vi "Refresh Display.vi"(6 "WaveformTemplate":waveform(dbl), 8 "error in":errorcluster, 9 "Temperature":dbl[](array[numeric]), 10 "Resistance":dbl[](array[numeric]), 11 "PRM in":refnum<class "PRM.lvclass">) -> (0 "error out":errorcluster, 2 "Measured":waveform(dbl)[](array[waveform]), 3 "PRM out":refnum<class "PRM.lvclass">)   [LabVIEW 2019, in "PRM.lvlib" / "PRM.lvclass"]
uses:
  Library/PRM.lvclass
  Library/PRM.lvclass/PRM.ctl
  builds/Instruments/Instruments.lvlibp/Library/Instruments.lvclass
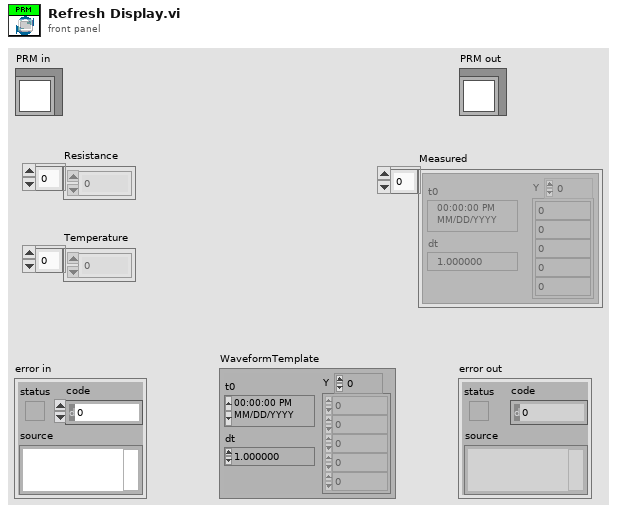
[diagram p1: front panel]
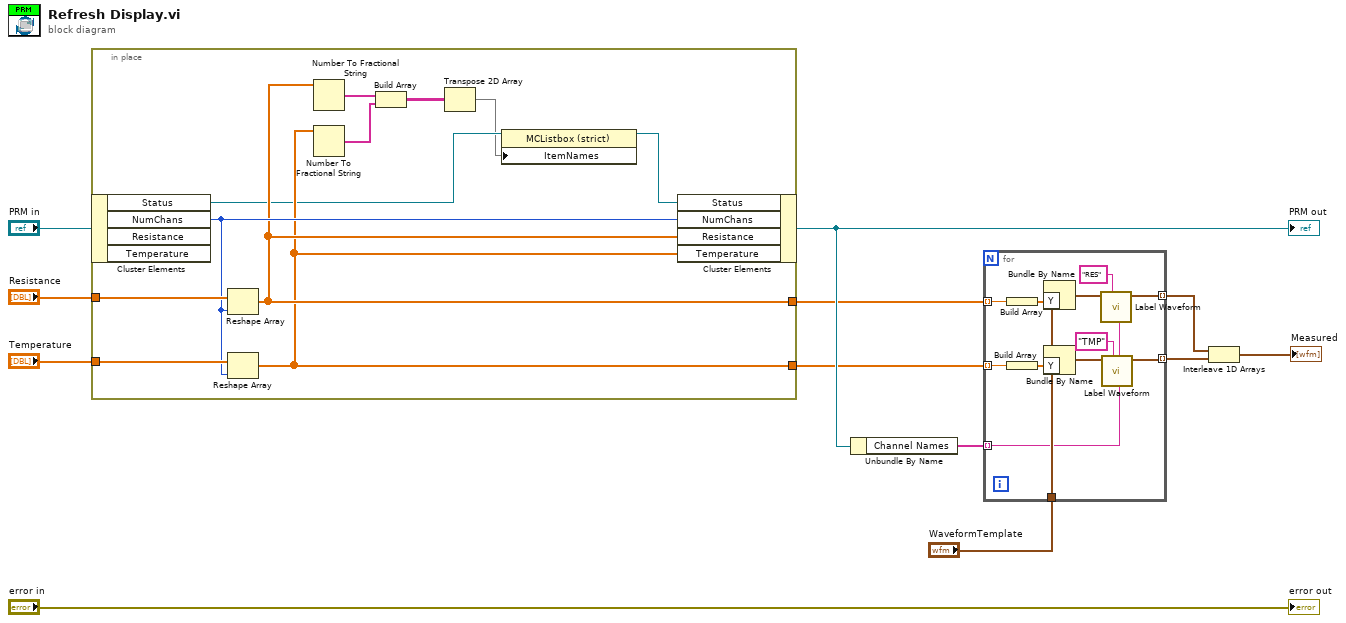
[diagram p0: block diagram]
diagram:
  n1 = in-place {
    in-place-border: "Resistance" -> [w23]
    in-place-border: "Temperature" -> [w22]
    in-place-border: [w20] -> w7
    in-place-border: [w19] -> w6
    n2 = in-place-cluster #1("PRM in") -> ("Status"=w16:refnum<vi>, "NumChans"=w21:i32)  [unwired: 2 out]
    n3 = Reshape Array(w23, w21) -> (w20:dbl[])
    n4 = Reshape Array(w22, w21) -> (w19:dbl[])
    n5 = Number To Fractional String(number=w20) -> (F-format string=w18:string[])  [unwired: 3 in]
    n6 = Number To Fractional String(number=w19) -> (F-format string=w17:string[])  [unwired: 3 in]
    n7 = Build Array(w18, w17) -> (w14:string[][])
    n8 = Transpose 2D Array(2D array=w14) -> (transposed array=w13:string[][])
    n9 = property class="MCListbox (strict)"(reference=w16, "ItemNames"=w13) -> (reference out=w15:refnum<vi>)  [unwired: 1 in, 1 out]
    n10 = in-place-cluster #1("Status"=w15, "NumChans"=w21, "Resistance"=w20, "Temperature"=w19) -> (w9:refnum<class "PRM.lvclass">)
  }
  "PRM out" <- w9
  n11 = Unbundle By Name(w9) -> ("Channel Names"=w8:string[])
  n12 = for {
    tunnel: w8 -> [w26] mode=indexing
    tunnel: w7 -> [w32] mode=indexing
    tunnel: w6 -> [w35] mode=indexing
    tunnel: "WaveformTemplate" -> [w31]
    tunnel: [w28] -> w3 mode=indexing
    tunnel: [w27] -> w2 mode=indexing
    n13 = Build Array(w32) -> (w33:dbl[])
    n14 = Build Array(w35) -> (w34:dbl[])
    n15 = Bundle By Name(cluster=w31, "Y"=w33) -> (w30:waveform(dbl))
    n16 = Bundle By Name(cluster=w31, "Y"=w34) -> (w29:waveform(dbl))
    n17 = call "Label Waveform.vi"("Unique Channel Name"=w26, "Measurement"="RES", "Input waveform"=w30) -> ("Labelled Waveform"=w28:waveform(dbl))  [unwired: 8 in]
    n18 = call "Label Waveform.vi"("Unique Channel Name"=w26, "Measurement"="TMP", "Input waveform"=w29) -> ("Labelled Waveform"=w27:waveform(dbl))  [unwired: 8 in]
  }
  n19 = Interleave 1D Arrays(w3, w2) -> (→"Measured":waveform(dbl)[])
  "error out" <- "error in"
